vi "Convert Data to View.vi"(7 "Display State In":T1={"Current Channels Info"=[], "Help Prefix"="", "Max Display Size"=8, "Max Size"=0, "Show Buttons"=TRUE, "Data Valid"=refnum, "Show Range"=FALSE, "Range Items"=[], "Range Index"=[]} caption="State", 11 "Channels Data":T7) -> (1 "Invalid Info":string, 2 "Data Valid?":bool, 3 "Channels View Out":T4[](array[typedef]))   [LabVIEW 2021, in "myRIO Channel List.xctl"]
uses:
  <vilib>/myRIO/Common/Express VI Framework/xctls/myRIO Channel List/myRIO Channel List.xctl
  <vilib>/myRIO/Common/Express VI Framework/xctls/myRIO Channel List/Data.ctl
  <vilib>/myRIO/Common/Express VI Framework/xctls/myRIO Channel List/typedefs/Channel Data.ctl
  <vilib>/myRIO/Common/Express VI Framework/xctls/myRIO Channel List/typedefs/Remove Channel.ctl
  <vilib>/myRIO/Common/Express VI Framework/xctls/myRIO Channel List/typedefs/Channel View.ctl
  <vilib>/myRIO/Common/Express VI Framework/xctls/myRIO Channel List/typedefs/Error Icon.ctl
  <vilib>/myRIO/Common/Express VI Framework/xctls/myRIO Channel List/State.ctl
  <vilib>/myRIO/Common/Profile Manager Framework/typedefs/Channel Info.ctl
  <vilib>/myRIO/Common/Express VI Framework/typedefs/Data Validate Ref.ctl
  <vilib>/myRIO/Common/Express VI Framework/vis/Express VI Framework Strings Global.vi
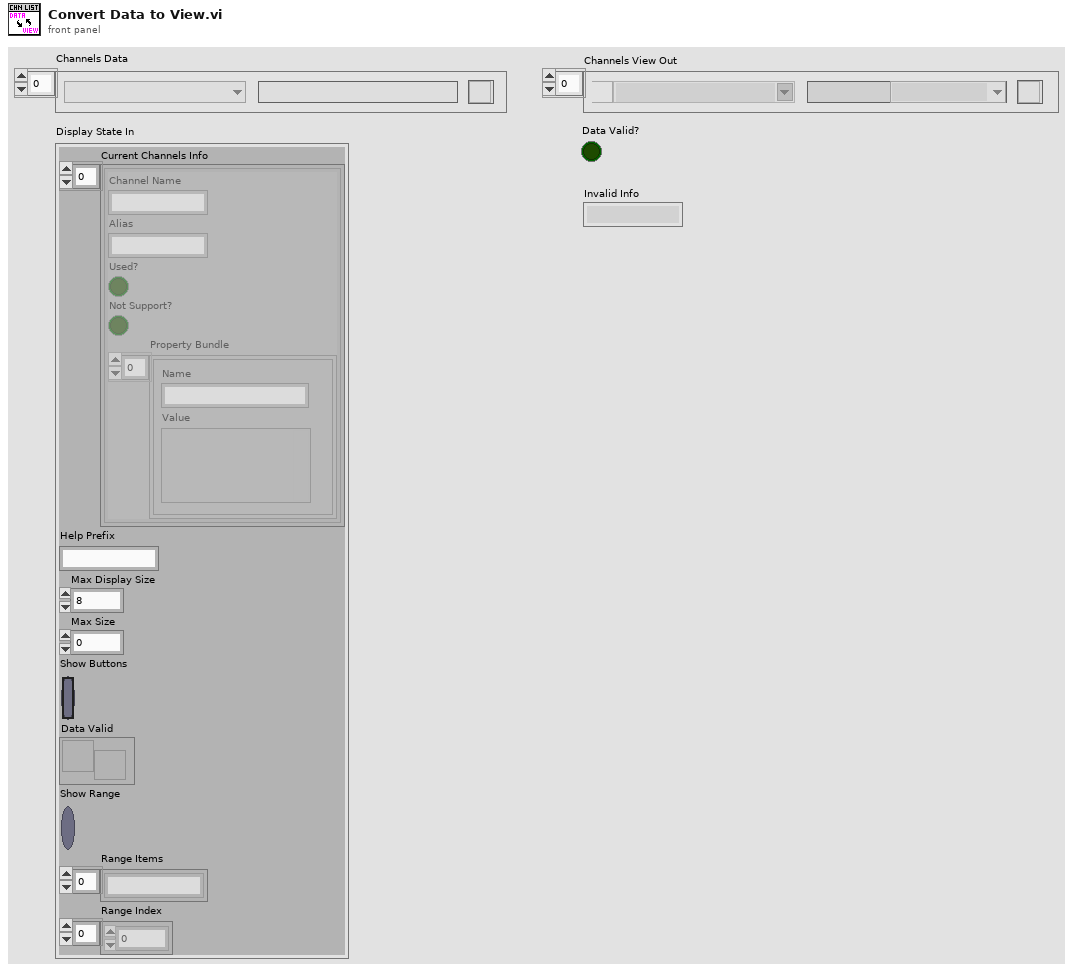
[diagram p1: front panel]
types:
  T1 = typedef "myRIO Channel List.xctl/State.ctl" = cluster{"Current Channels Info":T2[], "Help Prefix":string, "Max Display Size":i32, "Max Size":i32, "Show Buttons":bool, "Data Valid":T3, "Show Range":bool, "Range Items":string[], "Range Index":i32[]}
  T2 = typedef "Channel Info.ctl" = cluster{"Channel Name":string, "Alias":string, "Used?":bool, "Not Support?":bool, "Property Bundle":cluster{"Name":string, "Value":variant}[]}
  T3 = typedef "Data Validate Ref.ctl" = refnum<user-event>
  T4 = typedef "myRIO Channel List.xctl/Channel View.ctl" = cluster{"Error Icon":T5, "Channel Name":string, "Channel Alias":string, "Remove Channel":T6, "Index":i32, "Range":i32}
  T5 = typedef "myRIO Channel List.xctl/Error Icon.ctl" = bool
  T6 = typedef "myRIO Channel List.xctl/Remove Channel.ctl" = bool
  T7 = typedef "myRIO Channel List.xctl/Data.ctl" = T8[]
  T8 = typedef "myRIO Channel List.xctl/Channel Data.ctl" = cluster{"Channel Name":u16, "Channel Alias":string, "Remove Channel":T6, "Index":i32}
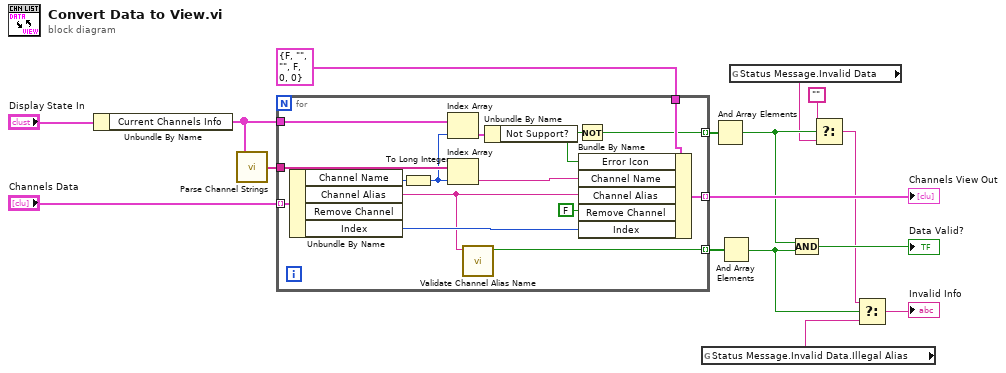
[diagram p0: block diagram]
diagram:
  n1 = Unbundle By Name("Display State In") -> ("Current Channels Info"=w11:T2[])
  n2 = call <vilib>:"Parse Channel Strings.vi"("Channels Info"=w11) -> ("Channel Strings"=w14:string[])
  n3 = for {
    tunnel: "Channels Data" -> [w31] mode=indexing
    tunnel: w14 -> [w29]
    tunnel: [w26] -> w12 mode=indexing
    tunnel: T4 {"Error Icon"=FALSE, "Channel Name"="", "Channel Alias"="", "Remove Channel"=FALSE, "Index"=0, "Range"=0} ("Channel") -> [w25]
    tunnel: w11 -> [w24]
    tunnel: [w19] -> w10 mode=indexing
    tunnel: [w17] -> w9 mode=indexing
    n4 = Unbundle By Name(w31) -> ("Channel Name"=w28:u16, "Channel Alias"=w18:string, "Index"=w30:i32)  [unwired: 1 out]
    n5 = To Long Integer(number=w28) -> (32bit integer=w23:i32)
    n6 = Index Array(array=w24, index=w23) -> (element=w22:T2)
    n7 = Index Array(array=w29, index=w23) -> (element=w27:string)
    n8 = call <vilib>:"Validate Channel Alias Name.vi"("Channel Alias"=w18) -> ("Valid?"=w17:bool)  [unwired: 9 in, 1 out]
    n9 = Unbundle By Name(w22) -> ("Not Support?"=w20:bool)
    n10 = Not(x=w20) -> (.not. x?=w19:bool)
    n11 = Bundle By Name(cluster=w25, "Error Icon"=w20, "Channel Name"=w27, "Channel Alias"=w18, "Remove Channel"=T6 FALSE, "Index"=w30) -> (w26:T4)
  }
  "Channels View Out" <- w12
  n12 = global read "Express VI Framework Strings Global.vi" "Status Message.Invalid Data.Illegal Alias"() -> (w1:string)
  n13 = And Array Elements(Boolean array=w10) -> (logical AND=w7:bool)
  n14 = And Array Elements(Boolean array=w9) -> (logical AND=w3:bool)
  n15 = global read "Express VI Framework Strings Global.vi" "Status Message.Invalid Data"() -> (w6:string)
  n16 = Compound Arithmetic op=AND(w7, w3) -> (→"Data Valid?":bool)
  n17 = Select(t="", s=w7, f=w6) -> (s? t:f=w2:string)
  n18 = Select(t=w2, s=w3, f=w1) -> (s? t:f=→"Invalid Info":string)
